vi "Wordle.vi"(11 "Submission LLB":path) -> (0 "error out":errorcluster, 2 "Test Summary":string, 3 "Score":T1)   [LabVIEW 2020]
uses:
  Valid Guesses--constant.vi
  <vilib>/AdvancedString/Delimited String to 1D String Array.vi
  <vilib>/Utility/error.llb/Error Cluster From Error Code.vi
panel:
  out "Current Solve":i32
  out "Elapsed Time":dbl
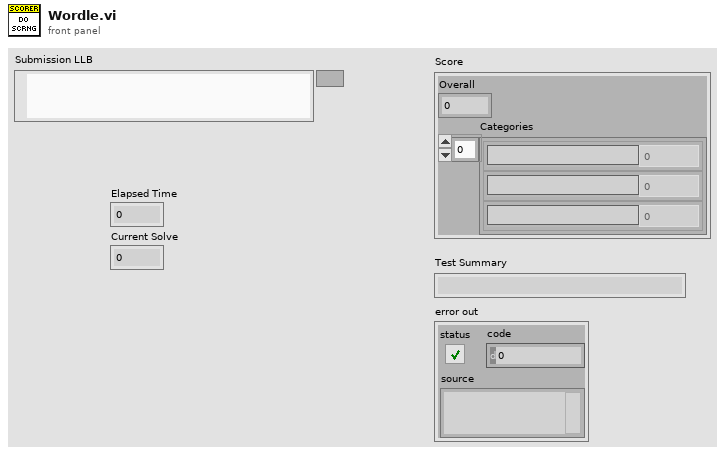
[diagram p1: front panel]
types:
  T1 = cluster{"Overall":dbl, "Categories":cluster{"Category":string, "Value":dbl}[]}
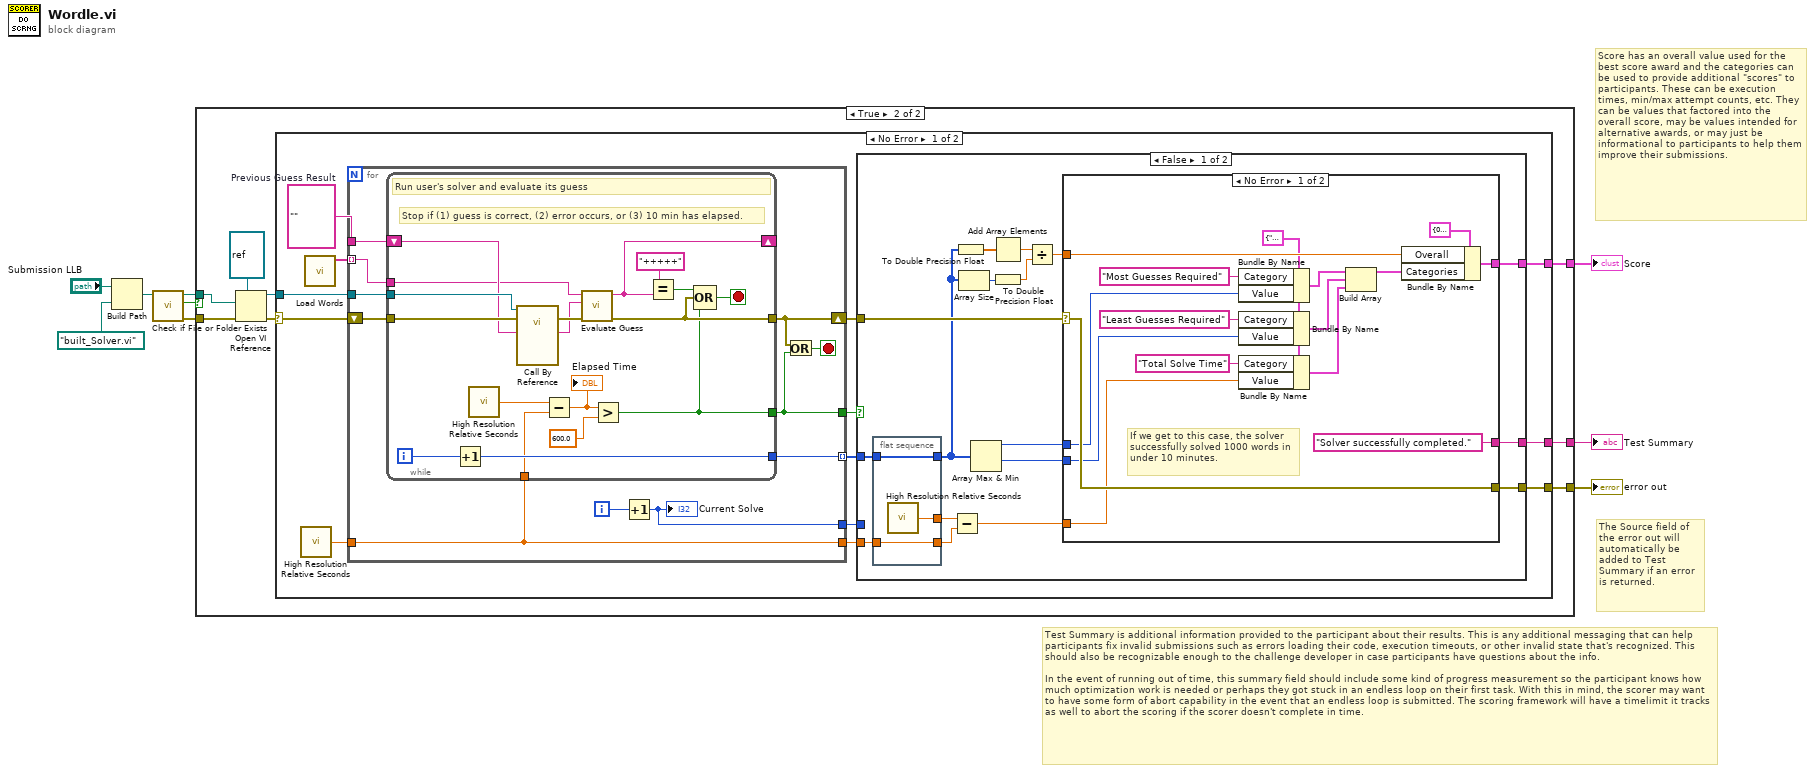
[diagram p0: block diagram]
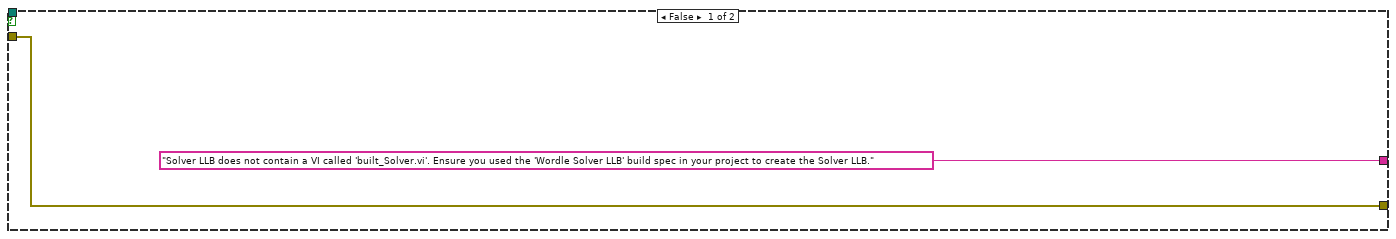
[diagram p2: hidden frame]
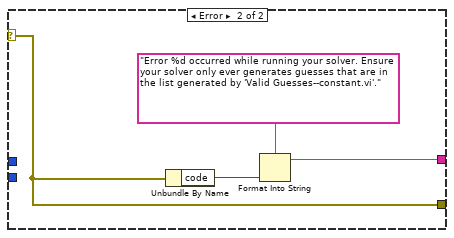
[diagram p3: hidden frame]
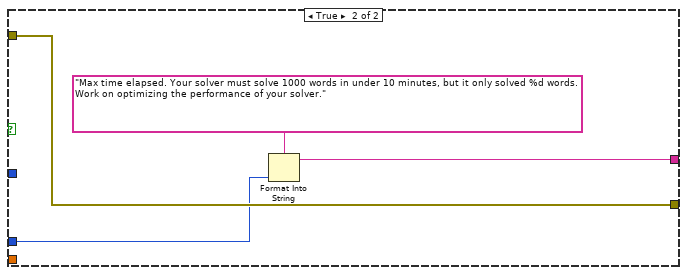
[diagram p4: hidden frame]
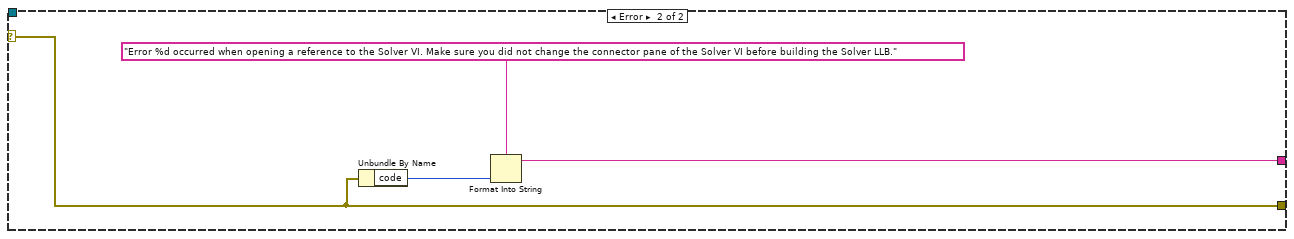
[diagram p5: hidden frame]
diagram:
  # "The Source field of the error out will automatically be added to Test Summary if an error is returned."
  # "Test Summary is additional information provided to the participant about their results. This is any additional messaging that can help participants fix invalid submissions such as errors loading their code, execution timeouts, or other invalid state that's recognized. This should also be recognizable enough to the challenge developer in case participants have questions about the info.\n\nIn the event of running out of time, this summary field should include some kind of progress measurement so the participant knows how much optimization work is needed or perhaps they got stuck in an endless loop on their first task. With this in mind, the scorer may want to have some form of abort capability in the event that an endless loop is submitted. The scoring framework will have a timelimit it tracks as well to abort the scoring if the scorer doesn't complete in time."
  # "Score has an overall value used for the best score award and the categories can be used to provide additional \"scores\" to participants. These can be execution times, min/max attempt counts, etc. They can be values that factored into the overall score, may be values intended for alternative awards, or may just be informational to participants to help them improve their submissions."
  n1 = Build Path(base path="Submission LLB", name or relative path=path "built_Solver.vi") -> (appended path=w7:path)
  n2 = call <vilib>:"Check if File or Folder Exists.vi"("path"=w7) -> ("error out"=w3:errorcluster, "file or folder exists?"=w5:bool, "dup path"=w6:path)  [unwired: 8 in]
  n3 = case shown="True" w5 {
    tunnel: w6 -> [_ w18]
    tunnel: [w11 w15] -> w4
    tunnel: w3 -> [w11 w19]
    tunnel: ["Solver LLB does not contain a VI called 'built_Solver.vi'. Ensure you used the 'Wordle Solver LLB' build spec in your project to create the Solver LLB." w13] -> w2
    tunnel: [_ w12] -> w1
    frame False {
    }
    frame True {
      n4 = Open VI Reference(type specifier VI Refnum (for type only)=refnum<vi> refnum, vi path=w18, error in (no error)=w19) -> (vi reference=w14:refnum<vi>, error out=w16:errorcluster)  [unwired: 3 in]
      n5 = case shown="No Error" w16 {
        selector: w16 -> [w32 w106]
        tunnel: [w25 w106] -> w15
        tunnel: w14 -> [w31 _]
        tunnel: [w24 w108] -> w13
        tunnel: [w23 _] -> w12
        frame No Error {
          w30 = ""  # Previous Guess Result
          n6 = call <vilib>:"High Resolution Relative Seconds.vi"() -> ("relative seconds"=w29:dbl)
          n7 = call "Load Words.vi"() -> ("Words"=w20:string[])  [unwired: 11 in]
          n8 = for {
            tunnel: w31 -> [w43]
            shift-right: [w41] -> w26
            shift-left: w32 -> [w42]
            tunnel: w20 -> [w39] mode=indexing
            tunnel: w30 -> [w38]
            tunnel: [w37] -> w27 mode=indexing
            tunnel: w29 -> [w36]
            tunnel: [w36] -> w28
            tunnel: [w34] -> w22
            tunnel: [w33] -> w21
            i -> [w40]
            stop <- w35 stop-if-true
            n9 = while {
              tunnel: w43 -> [w61]
              tunnel: w42 -> [w60]
              tunnel: [w52] -> w41
              shift-right: [w49] -> _
              shift-left: w38 -> [w59]
              tunnel: w39 -> [w51]
              tunnel: [w54] -> w37
              tunnel: w36 -> [w47]
              tunnel: [w44] -> w34
              i -> [w55]
              stop <- w58 stop-if-true
              # "Stop if (1) guess is correct, (2) error occurs, or (3) 10 min has elapsed."
              # "Run user's solver and evaluate its guess"
              n10 = Increment(x=w55) -> (x+1=w54:i32)
              n11 = call <vilib>:"High Resolution Relative Seconds.vi"() -> ("relative seconds"=w48:dbl)
              n12 = call-by-ref "?"(reference=w61, error in=w60, "Previous Guess Result"=w59) -> (error out=w53:errorcluster, "New Guess"=w50:string)  [unwired: 10 in, 1 out]
              n13 = Subtract(x=w48, y=w47) -> (x-y=w46:dbl)
              "Elapsed Time" <- w46
              n14 = call "Evaluate Guess.vi"("error in"=w53, "Guess"=w50, "Current Word"=w51) -> ("error out"=w52:errorcluster, "Result"=w49:string)  [unwired: 7 in]
              n15 = Greater?(x=w46, y=600.0) -> (0:w44:bool)
              n16 = Equal?(x="+++++", y=w49) -> (x = y?=w56:bool)
              n17 = Compound Arithmetic op=OR(w56, w52, w44) -> (w58:bool)
            }
            n18 = Increment(x=w40) -> (x+1=w33:i32)
            "Current Solve" <- w33
            n19 = Or(x=w41, y=w34) -> (x .or. y?=w35:bool)
          }
          n20 = case shown="False" w22 {
            tunnel: w28 -> [w78 _]
            tunnel: w27 -> [w68 _]
            tunnel: w26 -> [w75 w105]
            tunnel: [w74 w105] -> w25
            tunnel: [w73 w102] -> w24
            tunnel: [w72 _] -> w23
            tunnel: w21 -> [_ w103]
            frame False {
              n21 = flat-sequence {
                tunnel: [w101] -> w76
                tunnel: w78 -> [w101]
                tunnel: [w100] -> w77
                tunnel: w68 -> [w99]
                tunnel: [w99] -> w67
                frame #0 {
                  n22 = call <vilib>:"High Resolution Relative Seconds.vi"() -> ("relative seconds"=w100:dbl)
                }
              }
              n23 = Subtract(x=w77, y=w76) -> (x-y=w69:dbl)
              n24 = To Double Precision Float(number=w67) -> (double precision float=w66:dbl[])
              n25 = Array Size(array=w67) -> (size(s)=w64:i32)
              n26 = Array Max & Min(array=w67) -> (max value=w71:i32, min value=w70:i32)  [unwired: 2 out]
              n27 = Add Array Elements(numeric array=w66) -> (sum=w65:dbl)
              n28 = To Double Precision Float(number=w64) -> (double precision float=w63:dbl)
              n29 = Divide(x=w65, y=w63) -> (x/y=w62:dbl)
              n30 = case shown="No Error" w75 {
                selector: w75 -> [w94 w95]
                tunnel: [w94 w95] -> w74
                tunnel: ["Solver successfully completed." w97] -> w73
                tunnel: [w91 _] -> w72
                tunnel: w62 -> [w90 _]
                tunnel: w71 -> [w87 _]
                tunnel: w70 -> [w84 _]
                tunnel: w69 -> [w79 _]
                frame No Error {
                  w80 = cluster{"Category":string, "Value":dbl} {"Category"="", "Value"=0.0} ("Score Entry")
                  # "If we get to this case, the solver successfully solved 1000 words in under 10 minutes."
                  n31 = Bundle By Name(cluster=w80, "Category"="Most Guesses Required", "Value"=w87) -> (w85:cluster{"Category":string, "Value":dbl})
                  n32 = Bundle By Name(cluster=w80, "Category"="Least Guesses Required", "Value"=w84) -> (w83:cluster{"Category":string, "Value":dbl})
                  n33 = Bundle By Name(cluster=w80, "Category"="Total Solve Time", "Value"=w79) -> (w81:cluster{"Category":string, "Value":dbl})
                  n34 = Build Array(w85, w83, w81) -> (w89:cluster{"Category":string, "Value":dbl}[])
                  n35 = Bundle By Name(cluster=T1 {"Overall"=0.0, "Categories"=[]} ("Score"), "Overall"=w90, "Categories"=w89) -> (w91:T1)
                }
                frame Error {
                  n36 = Unbundle By Name(w95) -> ("code"=w96:i32)
                  n37 = Format Into String(format string="Error %d occurred while running your solver. Ensure your solver only ever generates guesses that are in the list generated by 'Valid Guesses--constant.vi'.", w96) -> (resulting string=w97:string)  [unwired: 2 in, 1 out]
                }
              }
            }
            frame True {
              n38 = Format Into String(format string="Max time elapsed. Your solver must solve 1000 words in under 10 minutes, but it only solved %d words. Work on optimizing the performance of your solver.", w103) -> (resulting string=w102:string)  [unwired: 2 in, 1 out]
            }
          }
        }
        frame Error {
          n39 = Unbundle By Name(w106) -> ("code"=w107:i32)
          n40 = Format Into String(format string="Error %d occurred when opening a reference to the Solver VI. Make sure you did not change the connector pane of the Solver VI before building the Solver LLB.", w107) -> (resulting string=w108:string)  [unwired: 2 in, 1 out]
        }
      }
    }
  }
  "Score" <- w1
  "Test Summary" <- w2
  "error out" <- w4
